vi "3.1.17-Decider Function.vi"() -> ()   [LabVIEW 2011]
uses:
  3.0 Flow Control/3.0 List of Loops.ctl
  4-High Neurons/4.1.2-Act Neuron TD.ctl
  3.0-Global.vi
  <vilib>/gmath/statdist.llb/Normal PDF.vi
  <vilib>/gmath/NI_Gmath.lvlib
panel:
  out "Waveform Graph":dbl[](graph)
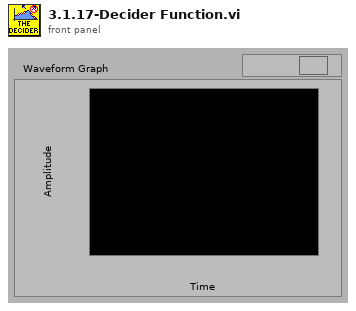
[diagram p1: front panel]
types:
  T1 = typedef "3.0 List of Loops.ctl" = enum16{"3.0 State Update", "3.0 GUI", "3.1 Act", "3.1 4.7.1 Act UDP", "3.1 Joystick", "3.2 Where", "3.2.0 Kalman Filter", "3.2 4.7.2 Where UDP", "3.3 What", "3.3 4.7.3 What UDP", "3.4 How", "3.4 4.7.4 How UDP", "3.5 Limbic", "3.8 TCP", "3.6 Cerebellum", "3.8 TCP Act", "3.11 Shallow Map", "3.1.17 Decider"}
  T2 = typedef "4.1.2-Act Neuron TD.ctl" = cluster{"Speed By Path":sgl[]}
  T3 = enum16{"Set Joystick", "Read Joystick", "Set Forebrain", "Read Forebrain", "Set Limbic", "Read Limbic", "Set Cerebellum", "Read Cerebellum", "Set Arbitrated", "Read Arbitrated", "Set LIDAR", "Read LIDAR", "Read Shallow Map", "Set Shallow Map", "Read Decider", "Set Decider"}
  T4 = typedef "4.2.0 Kalman State.ctl" = cluster{"X":dbl, "Y":dbl, "Theta":dbl, "V":dbl, "Omega":dbl, "Omega Dot":dbl}
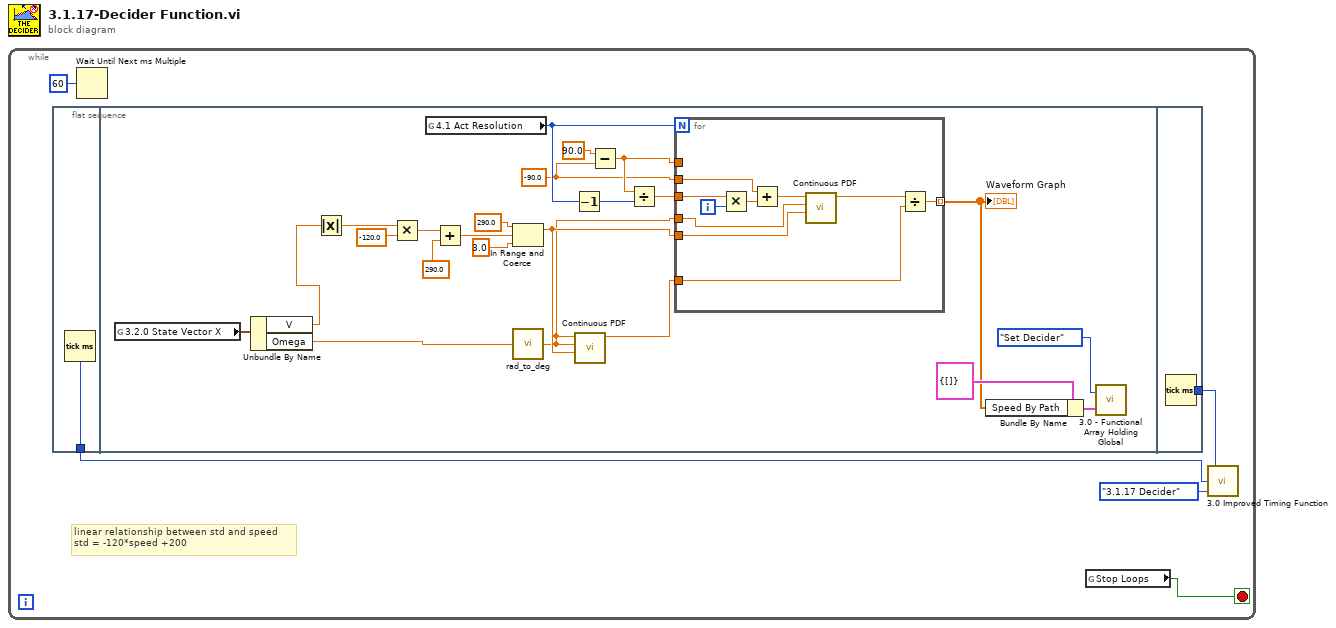
[diagram p0: block diagram]
diagram:
  n1 = while {
    stop <- w5 stop-if-true
    # "linear relationship between std and speed \nstd = -120*speed +200"
    n2 = flat-sequence {
      tunnel: [w6] -> w1
      tunnel: [w40] -> w2
      frame #0 {
        n3 = Tick Count (ms)() -> (millisecond timer value=w6:u32)
      }
      frame #1 {
        w21 = -90.0 ("Wheel Angle")
        n4 = global read "3.0-Global.vi" "3.2.0 State Vector X"() -> (w16:T4)
        n5 = Unbundle By Name(w16) -> ("V"=w7:dbl, "Omega"=w15:dbl)
        n6 = Absolute Value(x=w7) -> (abs(x)=w17:dbl)
        n7 = Multiply(x=w17, y=-120.0) -> (x*y=w23:dbl)
        n8 = global read "3.0-Global.vi" "4.1 Act Resolution"() -> (w28:u32)
        n9 = Add(x=w23, y=290.0) -> (x+y=w20:dbl)
        n10 = In Range and Coerce(upper limit=290.0, x=w20, lower limit=3.0) -> (coerced(x)=w14:dbl)  [unwired: 1 out]
        n11 = call "rad_to_deg.vi"("Radians"=w15) -> ("Degrees"=w13:dbl)
        n12 = Decrement(x=w28) -> (x-1=w27:u32)
        n13 = call-poly <vilib>:"Continuous PDF.vi"("std"=w14, "mean"=w13, "x"=w13) -> ("pdf(x)"=w12:dbl)  [unwired: 7 in, 1 out]
        n14 = Subtract(x=90.0 ("Wheel Angle"), y=w21) -> (x-y=w25:dbl)
        n15 = Divide(x=w25, y=w27) -> (x/y=w26:dbl)
        n16 = for {
          N: w28 -> [_]
          tunnel: w13 -> [w39]
          tunnel: w26 -> [w36]
          tunnel: w25 -> [_]
          tunnel: [w31] -> w9 mode=indexing
          tunnel: w14 -> [w34]
          tunnel: w21 -> [w32]
          tunnel: w12 -> [w30]
          i -> [w37]
          n17 = Multiply(x=w36, y=w37) -> (x*y=w38:dbl)
          n18 = Add(x=w32, y=w38) -> (x+y=w33:dbl)
          n19 = call-poly <vilib>:"Continuous PDF.vi"("std"=w34, "mean"=w39, "x"=w33) -> ("pdf(x)"=w35:dbl)  [unwired: 7 in, 1 out]
          n20 = Divide(x=w35, y=w30) -> (x/y=w31:dbl)
        }
        "Waveform Graph" <- w9
        n21 = Bundle By Name(cluster=T2 {"Speed By Path"=[]} ("Input Act Neurons"), "Speed By Path"=w9) -> (w8:T2)
        n22 = call "3.0 - Functional Array Holding Global.vi"("Input Act Neurons"=w8, "Mode"=T3."Set Decider") -> ()  [unwired: 1 out]
      }
      frame #2 {
        n23 = Tick Count (ms)() -> (millisecond timer value=w40:u32)
      }
    }
    n24 = Wait Until Next ms Multiple(millisecond multiple=u32 60) -> ()  [unwired: 1 out]
    n25 = global read "3.0-Global.vi" "Stop Loops"() -> (w5:bool)
    n26 = call "3.0 Improved Timing Function.vi"("Loop"=3.0_List_of_Loops."3.1.17 Decider", "Start"=w1, "End"=w2) -> ()  [unwired: 1 in]
  }
